vi "Test AMS Climate Chamber Template UI.vi"(10 "gRPC Port":i32, 11 "IP":string="localhost") -> ()   [LabVIEW 2023]
uses:
  <vilib>/ADAS Replay HIL/NodeGrpcService/NodeGrpcService_client/RPC Messages/adas_TimingSettings.ctl
  <vilib>/ADAS Replay HIL/NodeGrpcService/NodeGrpcService_client/RPC Messages/adas_PrioritySettings.ctl
  <vilib>/ADAS Replay HIL/NodeGrpcService/NodeGrpcService_client/RPC Messages/adas_TimePair.ctl
  <vilib>/ADAS Replay HIL/NodeGrpcService/NodeGrpcService_Client_Wrapper/NodeGrpcService_Client_Wrapper.lvlib
  Plugin/Custom gRPC/AMSClimateChamberTemplateService_Client_Wrapper/AMSClimateChamberTemplateService_Client_Wrapper.lvlib
  <vilib>/ADAS Replay HIL/NodeGrpcService/NodeGrpcService_client/NodeGrpcService_client.lvlib
panel:
  out "Loaded Version":string
  in  "Exit UI":bool
  out "error":errorcluster
  out "TimePair":T1
  out "Status":T2={"state"=enum."Running", "Cycle Max"=1000, "Cycle Min"=1000, "Exec Max"=3, "Exec Min"=2, "Idle Max"=994, "Idle Min"=992, "Wake Error Max"=2, "Wake Error Min"=2, "TX-RX Max"=0, "TX-RX Min"=0, "End-End Max"=0, "End-End Min"=0, "Output Error Max"=0, "Output Error Min"=0, "Priority Data"={"Priority"=100, "Processor"=-2}, "error"={"status"=FALSE, "code"=0}, "Custom 1"=0, "Custom 2"=0, "Custom 3"=0, "Custom 4"=0, "Custom 5"=0.0, "Custom 6"=0.0, "Custom 7"=0.0, "Custom 8"=0.0} {"Custom 8" format="%#_13g"}
  in  "Update SetNumber":bool
  in  "SetNumber":u32
  in  "Priority":T3
  in  "Timing":T4
  in  "Future Time Event (ns)":u64
  in  "Restart":bool
  in  "Update Priority":bool
  in  "Update Timing":bool
  in  "Reset Stats":bool
  in  "Pause":bool
  in  "Start":bool
  in  "Stop":bool
  # "Custom gRPC Code Testing:"
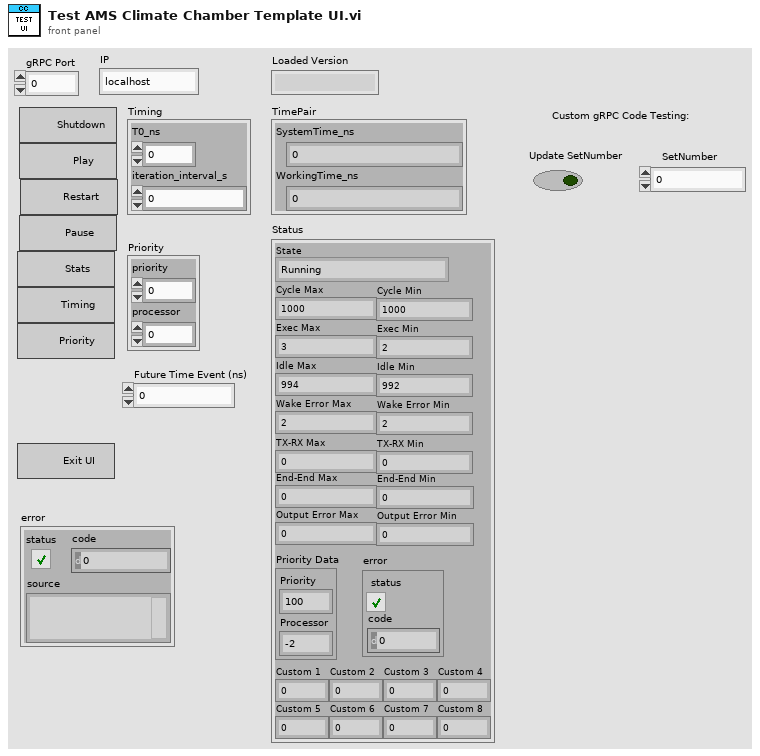
[diagram p1: front panel]
types:
  T1 = typedef "NodeGrpcService_client.lvlib/adas_TimePair.ctl" = cluster{"SystemTime_ns":u64, "WorkingTime_ns":u64}
  T2 = cluster{"state":enum32{"NotStarted", "Initialized", "Ready", "Running", "Shutdown"}, "Cycle Max":i32, "Cycle Min":i32, "Exec Max":i32, "Exec Min":i32, "Idle Max":i32, "Idle Min":i32, "Wake Error Max":i32, "Wake Error Min":i32, "TX-RX Max":i32, "TX-RX Min":i32, "End-End Max":i32, "End-End Min":i32, "Output Error Max":i32, "Output Error Min":i32, "Priority Data":cluster{"Priority":i32, "Processor":i32}, "error":cluster{"status":bool, "code":i32}, "Custom 1":u64, "Custom 2":u64, "Custom 3":u64, "Custom 4":u64, "Custom 5":dbl, "Custom 6":dbl, "Custom 7":dbl, "Custom 8":dbl}
  T3 = typedef "NodeGrpcService_client.lvlib/adas_PrioritySettings.ctl" = cluster{"priority":i64, "processor":i32}
  T4 = typedef "NodeGrpcService_client.lvlib/adas_TimingSettings.ctl" = cluster{"T0_ns":u64, "iteration_interval_s":dbl}
  T5 = typedef "grpc-lvsupport-release.lvlib/grpcId.ctl" = u64
  T6 = cluster{"SystemTime_ns":u64, "WorkingTime_ns":u64}
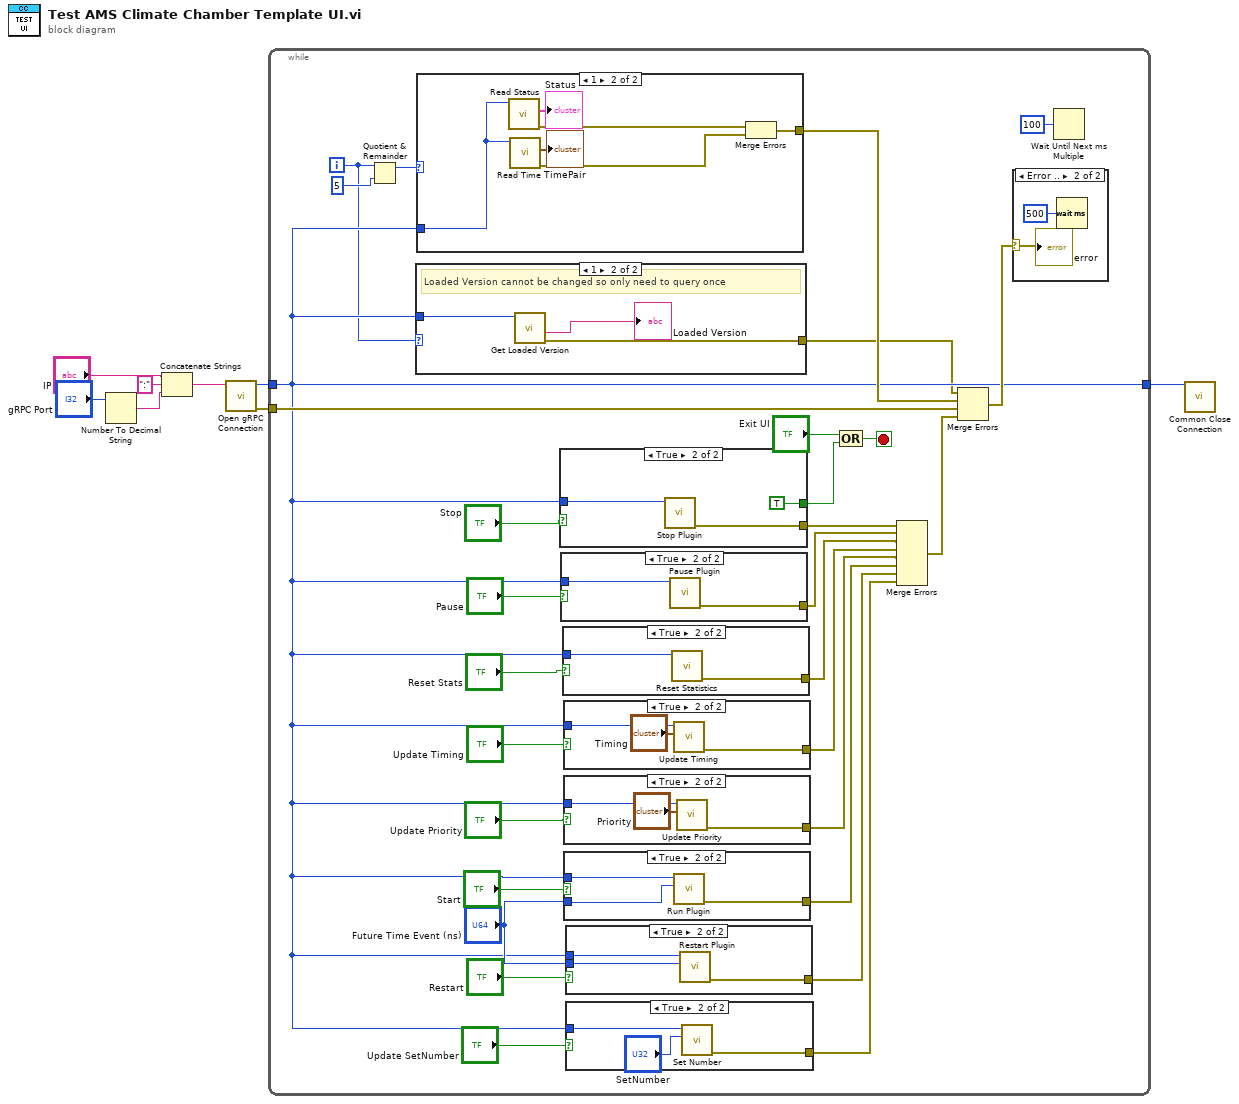
[diagram p0: block diagram]
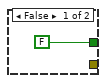
[diagram p10: hidden frame]
diagram:
  n1 = Number To Decimal String(number="gRPC Port") -> (decimal integer string=w8:string)  [unwired: 1 in]
  n2 = Concatenate Strings("IP", ":" ("string"), w8) -> (w1:string)
  n3 = call "Open gRPC Connection.vi"("address"=w1) -> ("error out"=w2:errorcluster, "gRPC ID Out"=w3:T5)  [unwired: 9 in]
  n4 = while {
    tunnel: w3 -> [w12]
    tunnel: w2 -> [w16]
    tunnel: [w12] -> w4
    i -> [w10]
    stop <- w13 stop-if-true
    n5 = Quotient & Remainder(x=w10, y=5) -> (x-y*floor(x/y)=w27:i32)  [unwired: 1 out]
    n6 = case shown="1" w10 {
      tunnel: w12 -> [_ w41]
      tunnel: [_ w39] -> w9
      frame Default {
      }
      frame 1 {
        # "Loaded Version cannot be changed so only need to query once"
        n7 = call <vilib>:"Get Loaded Version.vi"("gRPC ID"=w41) -> ("error out"=w39:errorcluster, "Version String"=→"Loaded Version":string)  [unwired: 7 in, 2 out]
      }
    }
    n8 = case shown="1" w27 {
      tunnel: w12 -> [_ w72]
      tunnel: [_ w67] -> w19
      frame 0, Default {
      }
      frame 1 {
        n9 = call <vilib>:"Read Status.vi"("gRPC ID"=w72) -> ("error out"=w69:errorcluster, "Status"=→"Status":T2)  [unwired: 7 in, 2 out]
        n10 = call <vilib>:"Read Time.vi"("gRPC ID"=w72) -> ("error out"=w68:errorcluster, "TimePair"=→"TimePair":T6)  [unwired: 8 in, 1 out]
        n11 = Merge Errors(w69, w68) -> (w67:errorcluster)
      }
    }
    n12 = case shown="True" "Stop" {
      tunnel: w12 -> [_ w64]
      tunnel: [_ w63] -> w26
      tunnel: [FALSE TRUE] -> w14
      frame False {
      }
      frame True {
        n13 = call <vilib>:"Stop Plugin.vi"("gRPC ID"=w64) -> ("error out"=w63:errorcluster)  [unwired: 8 in, 2 out]
      }
    }
    n14 = case shown="True" "Pause" {
      tunnel: w12 -> [_ w60]
      tunnel: [_ w59] -> w25
      frame False {
      }
      frame True {
        n15 = call <vilib>:"Pause Plugin.vi"("gRPC ID"=w60) -> ("error out"=w59:errorcluster)  [unwired: 8 in, 2 out]
      }
    }
    n16 = case shown="True" "Reset Stats" {
      tunnel: w12 -> [_ w58]
      tunnel: [_ w57] -> w24
      frame False {
      }
      frame True {
        n17 = call <vilib>:"Reset Statistics.vi"("gRPC ID"=w58) -> ("error out"=w57:errorcluster)  [unwired: 9 in, 1 out]
      }
    }
    n18 = case shown="True" "Update Timing" {
      tunnel: w12 -> [_ w56]
      tunnel: [_ w54] -> w23
      frame False {
      }
      frame True {
        n19 = call <vilib>:"Update Timing.vi"("Timing"="Timing", "gRPC ID"=w56) -> ("error out"=w54:errorcluster)  [unwired: 8 in, 1 out]
      }
    }
    n20 = case shown="True" "Update Priority" {
      tunnel: w12 -> [_ w53]
      tunnel: [_ w51] -> w22
      frame False {
      }
      frame True {
        n21 = call <vilib>:"Update Priority.vi"("Priority"="Priority", "gRPC ID"=w53) -> ("error out"=w51:errorcluster)  [unwired: 8 in, 1 out]
      }
    }
    n22 = case shown="True" "Start" {
      tunnel: w12 -> [_ w50]
      tunnel: "Future Time Event (ns)" -> [_ w49]
      tunnel: [_ w48] -> w21
      frame False {
      }
      frame True {
        n23 = call <vilib>:"Run Plugin.vi"("Future Time Event (ns)"=w49, "gRPC ID"=w50) -> ("error out"=w48:errorcluster)  [unwired: 7 in, 2 out]
      }
    }
    n24 = case shown="True" "Restart" {
      tunnel: w12 -> [_ w47]
      tunnel: "Future Time Event (ns)" -> [_ w46]
      tunnel: [_ w45] -> w20
      frame False {
      }
      frame True {
        n25 = call <vilib>:"Restart Plugin.vi"("Future Time Event (ns)"=w46, "gRPC ID"=w47) -> ("error out"=w45:errorcluster)  [unwired: 7 in, 2 out]
      }
    }
    n26 = case shown="True" "Update SetNumber" {
      tunnel: w12 -> [_ w44]
      tunnel: [_ w42] -> w11
      frame False {
      }
      frame True {
        n27 = call "Set Number.vi"("SetNumber"="SetNumber", "gRPC ID"=w44) -> ("error out"=w42:errorcluster)  [unwired: 8 in, 1 out]
      }
    }
    n28 = Compound Arithmetic op=OR("Exit UI", w14) -> (w13:bool)
    n29 = Merge Errors(w26, w25, w24, w23, w22, w21, w20, w11) -> (w18:errorcluster)
    n30 = Merge Errors(w9, w19, w16, w18) -> (w17:errorcluster)
    n31 = case shown="Error .." w17 {
      selector: w17 -> [_ w66]
      frame No Error {
      }
      frame Error {
        n32 = Wait (ms)(milliseconds to wait=u32 500) -> ()  [unwired: 1 out]
        "error" <- w66
      }
    }
    n33 = Wait Until Next ms Multiple(millisecond multiple=u32 100 ("milliseconds to wait")) -> ()  [unwired: 1 out]
  }
  n34 = call <vilib>:"Common Close Connection.vi"("gRPC ID"=w4) -> ()  [unwired: 10 in, 1 out]
